vi "TriggerTests_2.vi"() -> ()   [LabVIEW 2009]
uses:
  <vilib>/Utility/NIReport.llb/NI_report.lvclass
panel:
  in  "Test carac":bool
  in  "vclip":i32[](array[numeric])=[100, 100, 100, 100, 100, 100, 100, 100]
  in  "Voltages values":dbl[](array[numeric])=[0.05, 0.1, 0.2, 0.3, 0.4, 0.5, 0.6, 0.7, 0.8, 0.9, 1.0, 1.1, 1.2]
  in  "Channels values":i32[](array[numeric])=[0, 1, 2, 4, 5, 6]
  in  "Channels init":i32[](array[numeric])=[2100, 2100, 2100, 2100, 2100, 2100, 2100]
  in  "Test calib":bool
  in  "test2.5":bool=TRUE
  out "Att Calibration":dbl[](array[numeric])
  in  "test 2.3b":bool=TRUE
  in  "test 2.2":bool=TRUE
  out "minims":dbl[](array[numeric])
  in  "test 2.1":bool=TRUE
  in  "Instrument VISA in":T1={"AWG VISA"="81160A", "Oscilloscope  VISA "="DSO80204B", "Integration Board IP"="172.16.7.43", "connection ID"=refnum, "report out"=refnum, "report file path"=path "D:/CTA/LevelTriggerBoardTest/TestsData/sumtrigger_delay"}
  out "error out":errorcluster={"status"=TRUE, "code"=-1073807343, "source"="VISA Open in Agilent 81150.lvlib:Initialize.vi->instrumentsInitialization.vi->TriggerTests_2.vi"}
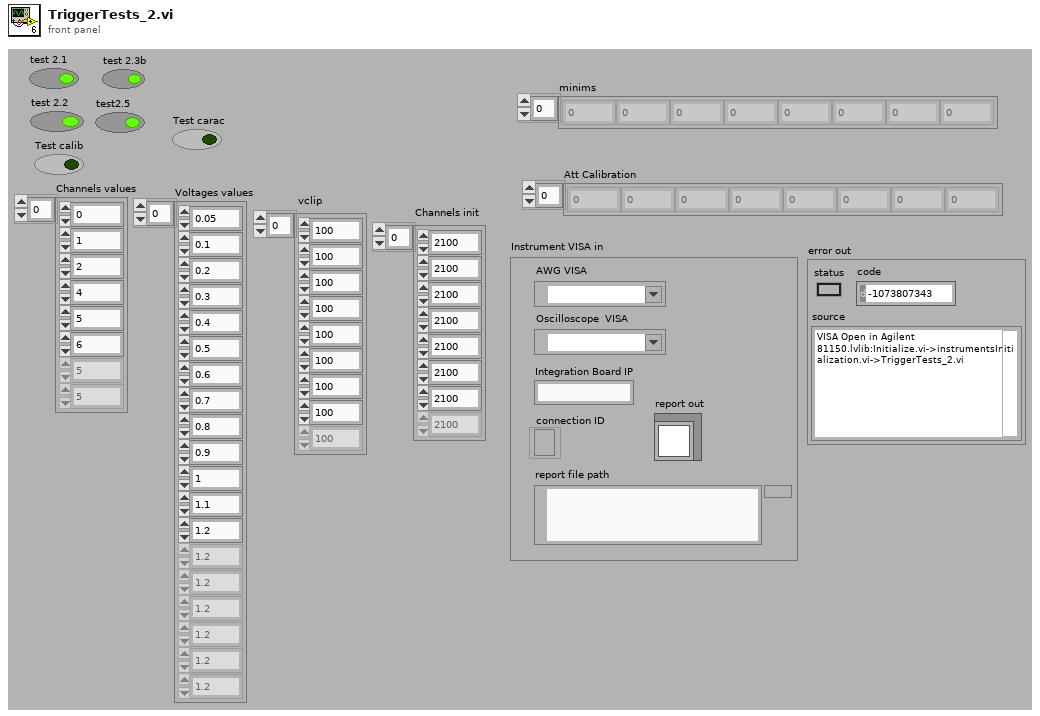
[diagram p1: front panel]
types:
  T1 = cluster{"AWG VISA":refnum<visa-resource-name>, "Oscilloscope  VISA ":refnum<visa-resource-name>, "Integration Board IP":string, "connection ID":refnum<k5>, "report out":refnum<class "NI_report.lvclass">, "report file path":path}
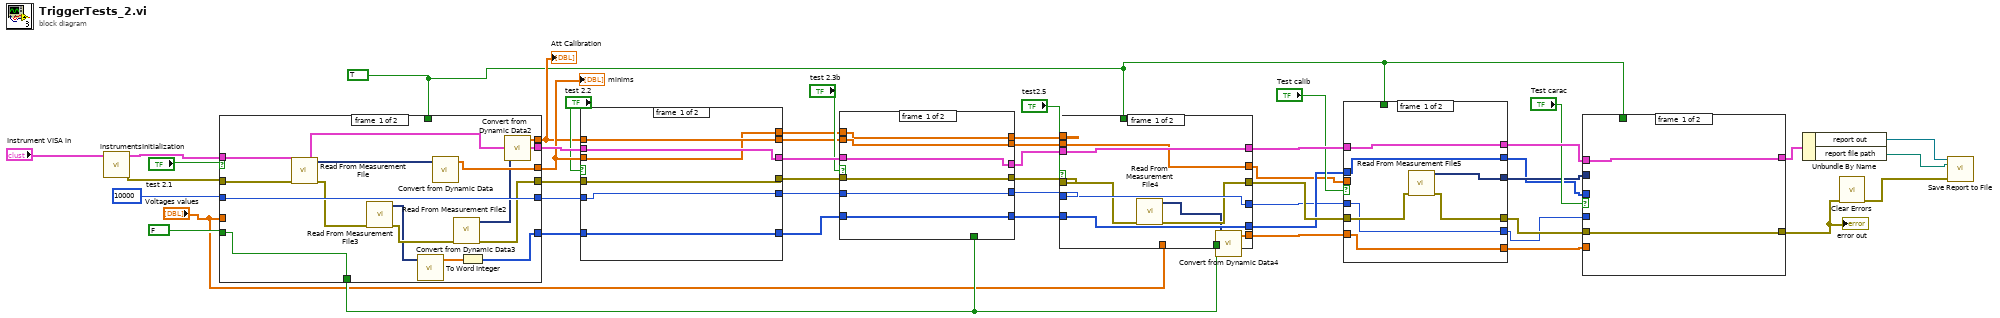
[diagram p0: block diagram]
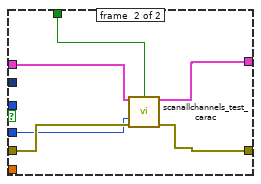
[diagram p2: hidden frame]
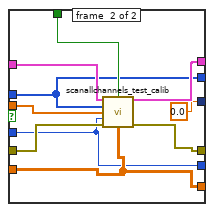
[diagram p3: hidden frame]
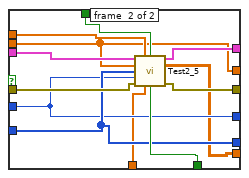
[diagram p4: hidden frame]
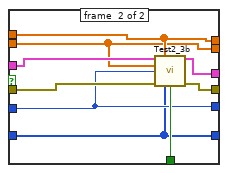
[diagram p5: hidden frame]
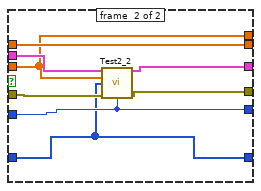
[diagram p6: hidden frame]
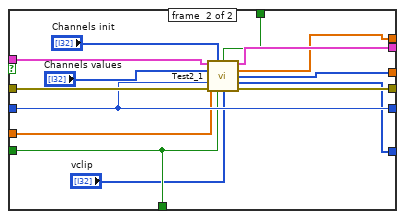
[diagram p7: hidden frame]
diagram:
  w1 = TRUE ("Report Enable")
  n1 = call "instrumentsInitialization.vi"("Instrument VISA in"="Instrument VISA in") -> ("error out"=w49:errorcluster, "Instrument VISA out"=w24:T1)  [unwired: 9 in]
  n2 = case shown="False" "test 2.1" {
    tunnel: w49 -> [w62 w77]
    tunnel: w24 -> [w63 w69]
    tunnel: 10000 ("Cycles Burst") -> [w59 w73]
    tunnel: [w58 w76] -> w47
    tunnel: [w63 w75] -> w45
    tunnel: [w60 w74] -> w44
    tunnel: [w59 w73] -> w42
    tunnel: [w56 w72] -> w34
    tunnel: [w55 w71] -> w28
    tunnel: FALSE ("L1 version") -> [w55 w71]
    tunnel: w1 -> [_ w70]
    tunnel: [w51 w68] -> w17
    tunnel: "Voltages values" -> [_ w64]
    frame #0 {
      n3 = call "Read From Measurement File"("error in (no error)"=w62) -> ("error out"=w53:errorcluster, "Signals"=w61:dynamicdata)  [unwired: 5 in, 4 out]
      n4 = call "Read From Measurement File3"("error in (no error)"=w53) -> ("error out"=w54:errorcluster, "Signals"=w52:dynamicdata)  [unwired: 5 in, 4 out]
      n5 = call "Convert from Dynamic Data3"("Dynamic Data Type"=w52) -> ("Array"=w50:dbl[])  [unwired: 3 in]
      n6 = call "Convert from Dynamic Data"("Dynamic Data Type"=w61) -> ("Array"=w60:dbl[])  [unwired: 3 in]
      n7 = call "Read From Measurement File2"("error in (no error)"=w54) -> ("error out"=w58:errorcluster, "Signals"=w57:dynamicdata)  [unwired: 5 in, 4 out]
      n8 = To Word Integer(number=w50) -> (16bit integer=w51:i16[])
      n9 = call "Convert from Dynamic Data2"("Dynamic Data Type"=w57) -> ("Array"=w56:dbl[])  [unwired: 3 in]
    }
    frame #1 {
      n10 = call "Test2_1.vi"("Instrument VISA in"=w69, "Channels init"="Channels init", "Report Enable"=w70, "Channels values"="Channels values", "Voltages values"=w64, "Cycles Burst"=w73, "error in"=w77, "L1 version"=w71, "vclip"="vclip") -> ("Instrument VISA out"=w75:T1, "Calibration"=w72:dbl[], "L1 min values"=w74:i32[], "Channels values"=w68:i32[], "error out"=w76:errorcluster)  [unwired: 2 in]
    }
  }
  "minims" <- w44
  "Att Calibration" <- w34
  n11 = case shown="False" "test 2.2" {
    tunnel: w47 -> [w81 w87]
    tunnel: w45 -> [w83 w90]
    tunnel: [w83 w89] -> w39
    tunnel: w44 -> [w79 w86]
    tunnel: w42 -> [w82 w85]
    tunnel: [w81 w88] -> w38
    tunnel: [w82 w85] -> w36
    tunnel: [w80 w91] -> w35
    tunnel: w34 -> [w80 w91]
    tunnel: [w79 w86] -> w32
    tunnel: w17 -> [w78 w84]
    tunnel: [w78 w84] -> w16
    frame #0 {
    }
    frame #1 {
      n12 = call "Test2_2.vi"("Instrument VISA in"=w90, "L1 min values"=w86, "channel array"=w84, "error in"=w87, "Cycles Burst"=w85) -> ("Instrument VISA out"=w89:T1, "error out"=w88:errorcluster)  [unwired: 7 in, 2 out]
    }
  }
  n13 = case shown="False" "test 2.3b" {
    tunnel: w39 -> [w97 w106]
    tunnel: [w97 w105] -> w30
    tunnel: [w96 w104] -> w31
    tunnel: w38 -> [w96 w103]
    tunnel: w36 -> [w95 w101]
    tunnel: w35 -> [w94 w99]
    tunnel: w28 -> [_ w102]
    tunnel: w32 -> [w93 w100]
    tunnel: [w95 w101] -> w29
    tunnel: [w93 w100] -> w27
    tunnel: [w94 w99] -> w26
    tunnel: w16 -> [w92 w98]
    tunnel: [w92 w98] -> w21
    frame #0 {
    }
    frame #1 {
      n14 = call "Test2_3b.vi"("Instrument VISA in"=w106, "Att minims"=w100, "Att Calibration ch"=w99, "Cycles Burst"=w101, "error in"=w103, "channel array"=w98, "L1 version"=w102) -> ("Instrument VISA out"=w105:T1, "error out"=w104:errorcluster)  [unwired: 5 in, 2 out]
    }
  }
  n15 = case shown="False" "test2.5" {
    tunnel: w30 -> [w114 w123]
    tunnel: [w114 w124] -> w19
    tunnel: [w109 w125] -> w20
    tunnel: w31 -> [w110 w126]
    tunnel: w29 -> [w111 w117]
    tunnel: w26 -> [w112 w118]
    tunnel: w28 -> [_ w121]
    tunnel: w27 -> [_ w120]
    tunnel: w1 -> [_ w122]
    tunnel: w21 -> [w113 w119]
    tunnel: [w113 w119] -> w15
    tunnel: [w112 w118] -> w14
    tunnel: [w111 w117] -> w13
    tunnel: [w107 w116] -> w12
    tunnel: "Voltages values" -> [_ w115]
    frame #0 {
      n16 = call "Read From Measurement File4"("error in (no error)"=w110) -> ("error out"=w109:errorcluster, "Signals"=w108:dynamicdata)  [unwired: 5 in, 4 out]
      n17 = call "Convert from Dynamic Data4"("Dynamic Data Type"=w108) -> ("Array"=w107:dbl[][])  [unwired: 3 in]
    }
    frame #1 {
      n18 = call "Test2_5.vi"("Instrument VISA in"=w123, "Att minims"=w120, "Report Enable"=w122, "Att Calibration"=w118, "channels"=w119, "Cycles Burst"=w117, "error in"=w126, "voltages"=w115, "L1 version"=w121) -> ("Instrument VISA out"=w124:T1, "Clipping"=w116:dbl[][], "error out"=w125:errorcluster)  [unwired: 3 in, 1 out]
    }
  }
  n19 = case shown="False" "Test calib" {
    tunnel: [w130 w139] -> w9
    tunnel: w20 -> [w131 w140]
    tunnel: [w133 w142] -> w8
    tunnel: w19 -> [w133 w141]
    tunnel: w1 -> [_ w143]
    tunnel: w15 -> [w128 w135]
    tunnel: w14 -> [_ w138]
    tunnel: w13 -> [w127 w134]
    tunnel: w12 -> [w129 w136]
    tunnel: [w132 0.0] -> w5
    tunnel: [w129 w136] -> w4
    tunnel: [w128 w135] -> w3
    tunnel: [w127 w134] -> w2
    frame #0 {
      n20 = call "Read From Measurement File5"("error in (no error)"=w131) -> ("error out"=w130:errorcluster, "Signals"=w132:dynamicdata)  [unwired: 5 in, 4 out]
    }
    frame #1 {
      n21 = call "scanallchannels_test_calib.vi"("Instrument VISA in"=w141, "Save test data"=w143, "Channels values"=w135, "Channels init"=w138, "Cycles Burst"=w134, "error in"=w140, "Clipping"=w136) -> ("Instrument VISA out"=w142:T1, "error out"=w139:errorcluster)  [unwired: 6 in, 1 out]
    }
  }
  n22 = case shown="True" "Test carac" {
    tunnel: [w145 w147] -> w10
    tunnel: w9 -> [w145 w148]
    tunnel: [w144 w150] -> w7
    tunnel: w8 -> [w144 w149]
    tunnel: w1 -> [_ w151]
    tunnel: w3 -> [_ _]
    tunnel: w2 -> [_ w146]
    tunnel: w4 -> [_ _]
    tunnel: w5 -> [_ _]
    frame #0 {
    }
    frame #1 {
      n23 = call "scanallchannels_test_carac.vi"("Instrument VISA in"=w149, "Save test data"=w151, "Cycles Burst"=w146, "error in"=w148) -> ("Instrument VISA out"=w150:T1, "error out"=w147:errorcluster)  [unwired: 9 in, 1 out]
    }
  }
  "error out" <- w10
  n24 = Unbundle By Name(w7) -> ("report out"=w48:refnum<class "NI_report.lvclass">, "report file path"=w22:path)
  n25 = call <vilib>:"Clear Errors.vi"("error in (no error)"=w10) -> ("error out"=w41:errorcluster)  [unwired: 6 in]
  n26 = call-dynamic "Save Report to File.vi"("report in"=w48, "report file path"=w22, "error in (no error)"=w41) -> ()  [unwired: 11 in, 2 out]
